vi "Correction factor to PSA.vi"(6 "Type of factor":u16(ring) items=["Antenna", "Cable", "Other", "User"], 7 "Input Array":dbl[][](array[numeric]), 8 "error in (no error)":errorcluster, 9 "Number of Columns":i32=2, 10 "Number of Rows":i32=9, 11 "VISA in":refnum<visa-resource-name>) -> (0 "VISA out":refnum<visa-resource-name>, 1 "Status Indicator":T1, 2 "Numeric":dbl format="%#_13g", 3 "Resulting string":string)   [LabVIEW 2016]
doc: "Write SCPI command to PSA to setup correction factor."
panel:
  out "error out":errorcluster
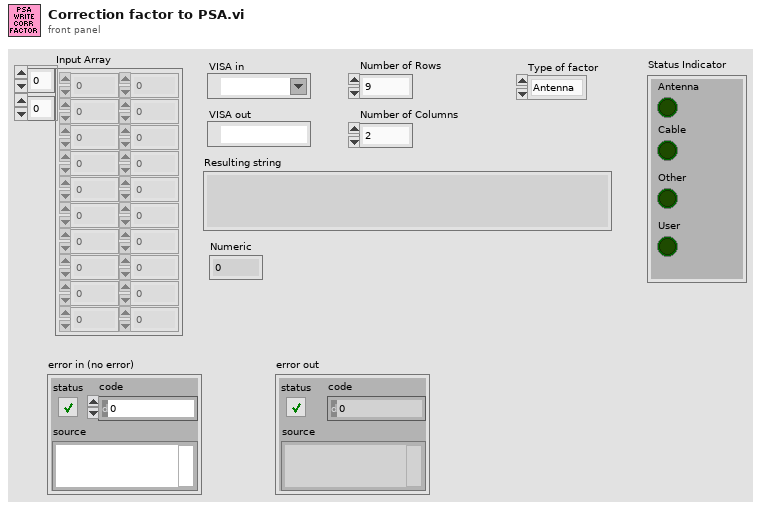
[diagram p1: front panel]
types:
  T1 = cluster{"Antenna":bool, "Cable":bool, "Other":bool, "User":bool}
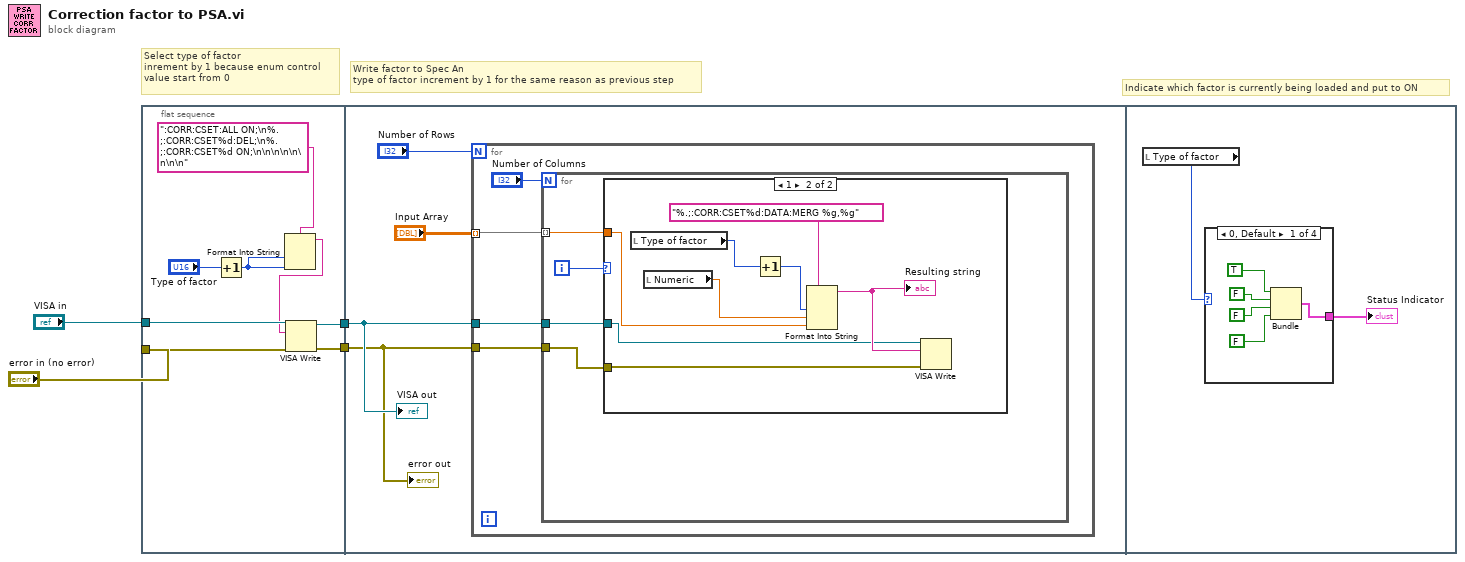
[diagram p0: block diagram]
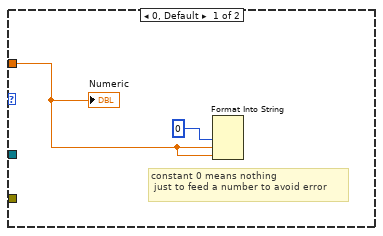
[diagram p2: hidden frame]
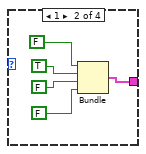
[diagram p3: hidden frame]
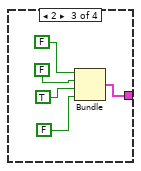
[diagram p4: hidden frame]
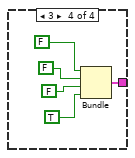
[diagram p5: hidden frame]
diagram:
  # "Indicate which factor is currently being loaded and put to ON"
  # "Write factor to Spec An\ntype of factor increment by 1 for the same reason as previous step"
  # "Select type of factor\ninrement by 1 because enum control\nvalue start from 0"
  n1 = flat-sequence {
    tunnel: [w12] -> w4
    tunnel: [w11] -> w3
    tunnel: "VISA in" -> [w9]
    tunnel: "error in (no error)" -> [w10]
    tunnel: w4 -> [w15]
    tunnel: w3 -> [w13]
    frame #0 {
      n2 = Increment(x="Type of factor") -> (x+1=w6:u16)
      n3 = Format Into String(format string=":CORR:CSET:ALL ON;\n%.;:CORR:CSET%d:DEL;\n%.;:CORR:CSET%d ON;\n\n\n\n\n\n\n\n", w6, w6) -> (resulting string=w7:string)  [unwired: 2 in, 1 out]
      n4 = VISA Write(VISA resource name=w9, write buffer=w7, error in (no error)=w10) -> (VISA resource name out=w12:refnum<visa-resource-name>, error out=w11:errorcluster)  [unwired: 1 out]
    }
    frame #1 {
      n5 = for {
        N: "Number of Rows" -> [_]
        tunnel: "Input Array" -> [w19] mode=indexing
        tunnel: w15 -> [w18]
        tunnel: w13 -> [w17]
        n6 = for {
          N: "Number of Columns" -> [_]
          tunnel: w19 -> [w23] mode=indexing
          tunnel: w18 -> [w22]
          tunnel: w17 -> [w21]
          i -> [w24]
          n7 = case shown="1" w24 {
            tunnel: w23 -> [w26 w29]
            tunnel: w22 -> [_ w32]
            tunnel: w21 -> [_ w31]
            frame 0, Default {
              # "constant 0 means nothing\n just to feed a number to avoid error"
              n8 = Format Into String(u16 0 ("input 1"), w26, w26) -> ()  [unwired: 3 in, 2 out]
              "Numeric" <- w26
            }
            frame 1 {
              n9 = local read "Type of factor"() -> (w28:u16)
              n10 = local read "Numeric"() -> (w30:dbl)
              n11 = Increment(x=w28) -> (x+1=w27:u16)
              n12 = Format Into String(format string="%.;:CORR:CSET%d:DATA:MERG %g,%g", w27, w30, w29) -> (resulting string=w33:string)  [unwired: 2 in, 1 out]
              "Resulting string" <- w33
              n13 = VISA Write(VISA resource name=w32, write buffer=w33, error in (no error)=w31) -> ()  [unwired: 3 out]
            }
          }
        }
      }
      "VISA out" <- w15
      "error out" <- w13
    }
    frame #2 {
      n14 = local read "Type of factor"() -> (w36:u16)
      n15 = case shown="0, Default" w36 {
        tunnel: [w37 w42 w47 w52] -> w35
        frame 0, Default {
          n16 = Bundle(TRUE, FALSE, FALSE, FALSE) -> (w37:cluster{bool, bool, bool, bool})  [unwired: 1 in]
        }
        frame 1 {
          n17 = Bundle(FALSE, TRUE, FALSE, FALSE) -> (w42:cluster{bool, bool, bool, bool})  [unwired: 1 in]
        }
        frame 2 {
          n18 = Bundle(FALSE, FALSE, TRUE, FALSE) -> (w47:cluster{bool, bool, bool, bool})  [unwired: 1 in]
        }
        frame 3 {
          n19 = Bundle(FALSE, FALSE, FALSE, TRUE) -> (w52:cluster{bool, bool, bool, bool})  [unwired: 1 in]
        }
      }
      "Status Indicator" <- w35
    }
  }
